vi "坐标转索引.vi"(10 "图形程序":refnum<vi>, 11 "坐标":T1) -> (3 "索引":cluster{"列":i32, "行":i32})   [LabVIEW 2020]
uses:
  <vilib>/Utility/miscctls.llb/LVPoint32TypeDef.ctl
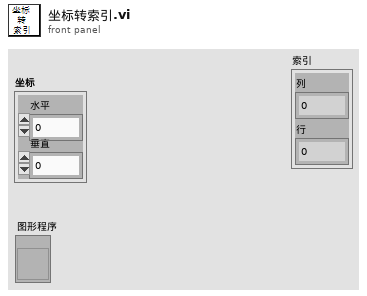
[diagram p1: front panel]
types:
  T1 = typedef "LVPoint32TypeDef.ctl" = cluster{"Horizontal":i32, "Vertical":i32}
  T2 = typedef "LVPositionTypeDef.ctl" = cluster{"Left":i32, "Top":i32}
  T3 = typedef "LVBoundsTypeDef.ctl" = cluster{"Width":u32, "Height":u32}
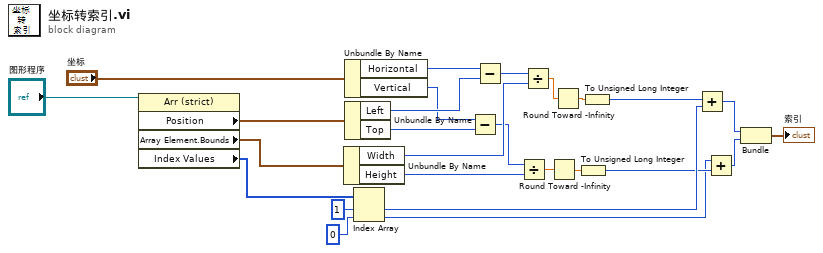
[diagram p0: block diagram]
diagram:
  n1 = property class="Arr (strict)"(reference="图形程序") -> ("Position"=w4:T2, "Array Element.Bounds"=w6:T3, "Index Values"=w5:u32[])  [unwired: 1 in, 2 out]
  n2 = Unbundle By Name(w6) -> ("Width"=w23:u32, "Height"=w19:u32)
  n3 = Unbundle By Name("坐标") -> ("Horizontal"=w26:i32, "Vertical"=w21:i32)
  n4 = Unbundle By Name(w4) -> ("Left"=w25:i32, "Top"=w20:i32)
  n5 = Index Array(array=w5, index #1=1 ("索引"), index #2=0 ("索引")) -> (element #1=w12:u32, element #2=w10:u32)
  n6 = Subtract(x=w21, y=w20) -> (x-y=w22:i32)
  n7 = Subtract(x=w26, y=w25) -> (x-y=w24:i32)
  n8 = Divide(x=w22, y=w19) -> (x/y=w17:dbl)
  n9 = Divide(x=w24, y=w23) -> (x/y=w18:dbl)
  n10 = Round Toward -Infinity(1:w17) -> (0:w15:dbl)
  n11 = Round Toward -Infinity(1:w18) -> (0:w16:dbl)
  n12 = To Unsigned Long Integer(number=w15) -> (unsigned 32bit integer=w11:u32)
  n13 = To Unsigned Long Integer(number=w16) -> (unsigned 32bit integer=w13:u32)
  n14 = Add(x=w13, y=w12) -> (x+y=w8:u32)
  n15 = Add(x=w10, y=w11) -> (x+y=w7:u32)
  n16 = Bundle(w8, w7) -> (→"索引":cluster{u32, u32})  [unwired: 1 in]
